vi "Create Settings Item.vi"(8 "error in (no error)":errorcluster) -> (0 "error out":errorcluster, 3 "Settings out":refnum<class "Settings.lvclass">)   [LabVIEW 2015, in "Item Actor.lvlib" / "Settings.lvclass"]
uses:
  Settings.lvclass
  <vilib>/picture/picture.llb/imagedata.ctl
  Generic Item/Generic Item.lvclass/Generic Item.ctl
  Generic Item/Write Weight.vi
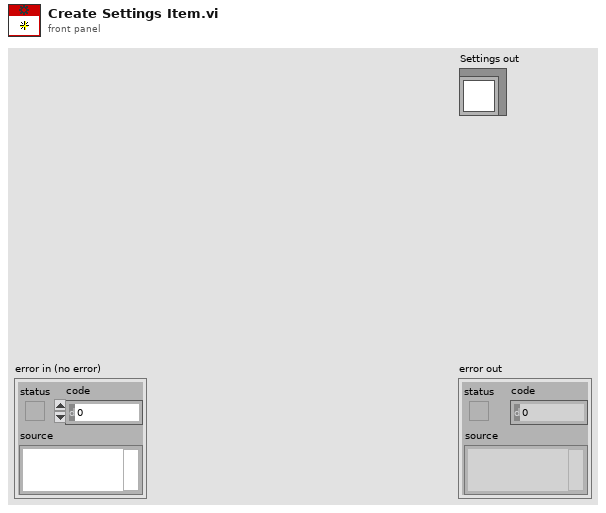
[diagram p1: front panel]
types:
  T1 = typedef "imagedata.ctl" = cluster{"image type":i32, "image depth":i32, "image":u8[], "mask":u8[], "colors":u32[], "Rectangle":cluster{"left":i16, "top":i16, "right":i16, "bottom":i16}}
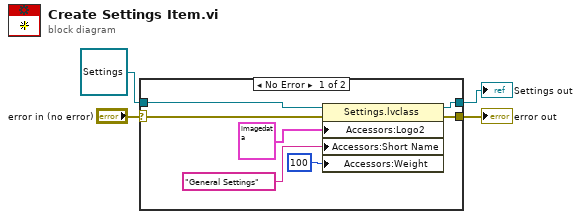
[diagram p0: block diagram]
diagram:
  n1 = case shown="No Error" "error in (no error)" {
    selector: "error in (no error)" -> [w7 w13]
    tunnel: [w6 w13] -> w3
    tunnel: [w8 w12] -> w1
    tunnel: refnum<class "Settings.lvclass"> refnum ("Settings in") -> [w11 w12]
    frame No Error {
      n2 = property class="Settings.lvclass"(reference=w11, error in=w7, "Accessors:Logo2"=T1 {"image type"=0, "image depth"=32, "image"=array[16384 elements], "mask"=[0, 0, 0, 0, 0, 0, 0, 0, 0, 0, 0, 0, 0, 120, 14, 0, 0, 0, 0, 0, 0, 248, 31, 0, 0, 0, 0, 0, 0, 124, 31, 0, 0, 0, 0, 0, 0, 127, 255, 0, 0, 0, 0, 0, 0, 127, 254, 0, 0, 0, 0, 0, 0, 127, 254, 0, 0, 0, 0, 0, 0, 255, 255, 0, 0, 0, 0, 0, 49, 255, 255, 140, 0, 0, 0, 0, 127, 255, 255, 254, 0, 0, 0, 0, 127, 255, 255, 254, 0, 0, 0, 0, 127, 248, 31, 254, 0, 0, 0, 0, 63, 240, 15, 252, 0, 0, 0, 0, 31, 224, 7, 248, 0, 0, 0, 0, 15, 224, 7, 240, 0, 0, 0, 0, 15, 224, 3, 240, 0, 0, 0, 0, 15, 224, 3, 240, 0, 0, 0, 0, 15, 224, 7, 240, 0, 0, 0, 0, 31, 224, 7, 248, 0, 0, 0, 0, 63, 240, 15, 252, 0, 0, 0, 0, 127, 248, 31, 254, 0, 0, 0, 0, 127, 254, 127, 254, 0, 0, 62, 0, 127, 255, 255, 254, 0, 0, 63, 0, 49, 255, 255, 140, 0, 0, 63, 0, 0, 255, 255, 0, 0, 0, 63, 0, 0, 127, 254, 0, 0, 0, 63, 0, 0, 127, 254, 0, 1, 128, 127, 0, 224, 127, 254, 0, 3, 224, 127, 129, 240, 252, 63, 0, 7, 243, 255, 227, 248, 248, 31, 0, 7, 255, 255, 255, 248, 112, 14, 0, 7, 255, 255, 255, 248, 0, 0, 0, 3, 255, 255, 255, 240, 0, 0, 0, 1, 255, 255, 255, 224, 0, 0, 0, 1, 255, 255, 255, 224, 0, 0, 0, 0, 255, 255, 255, 192, 0, 0, 0, 1, 255, 192, 255, 192, 0, 0, 0, 1, 255, 0, 127, 224, 0, 0, 0, 3, 254, 0, 63, 224, 0, 0, 0, 3, 254, 0, 31, 240, 0, 0, 0, 255, 252, 0, 15, 255, 128, 0, 0, 255, 252, 0, 15, 255, 192, 0, 0, 255, 252, 0, 15, 255, 192, 0, 0, 255, 252, 0, 15, 255, 192, 0, 0, 255, 252, 0, 15, 255, 192, 0, 0, 255, 252, 0, 15, 255, 192, 0, 0, 15, 252, 0, 31, 252, 0, 0, 0, 3, 254, 0, 31, 224, 0, 0, 0, 1, 255, 0, 63, 224, 0, 0, 0, 1, 255, 128, 255, 224, 0, 0, 0, 0, 255, 255, 255, 192, 0, 0, 0, 0, 255, 255, 255, 192, 0, 0, 0, 1, 255, 255, 255, 224, 0, 0, 0, 3, 255, 255, 255, 240, 0, 0, 0, 7, 255, 255, 255, 240, 0, 0, 0, 7, 255, 255, 255, 248, 0, 0, 0, 7, 251, 255, 247, 248, 0, 0, 0, 3, 224, 255, 193, 240, 0, 0, 0, 1, 192, 127, 0, 224, 0, 0, 0, 0, 0, 127, 0, 0, 0, 0, 0, 0, 0, 63, 0, 0, 0, 0, 0, 0, 0, 63, 0, 0, 0, 0, 0, 0, 0, 63, 0, 0, 0, 0, 0, 0, 0, 63, 0, 0, 0, 0, 0], "colors"=[], "Rectangle"={"left"=0, "top"=0, "right"=64, "bottom"=64}} ("image data"), "Accessors:Short Name"="General Settings" ("Short Name"), "Accessors:Weight"=100 ("Weight")) -> (reference out=w8:refnum<class "Settings.lvclass">, error out=w6:errorcluster)
    }
    frame Error {
    }
  }
  "error out" <- w3
  "Settings out" <- w1
